vi "Read.vi"(8 "error in (no error)":errorcluster, 10 "count":i32, 11 "Stream Upload Controller in":refnum<class "Stream Upload Controller.lvclass">) -> (0 "error out":errorcluster, 2 "data":u8[](array[numeric]), 3 "Stream Upload Controller out":refnum<class "Stream Upload Controller.lvclass">)   [LabVIEW 2020, in "NI_SFTP.lvlib" / "Stream Upload Controller.lvclass"]
uses:
  <vilib>/net/SFTP/API/Support/Upload/Stream/Stream Upload Controller.lvclass
  <vilib>/net/SFTP/API/Support/Upload/Stream/Stream Upload Controller.lvclass/Stream Upload Controller.ctl
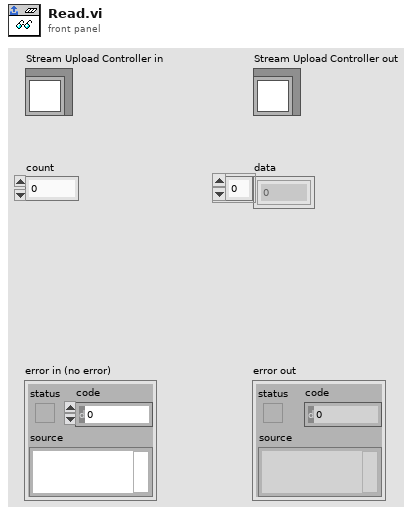
[diagram p1: front panel]
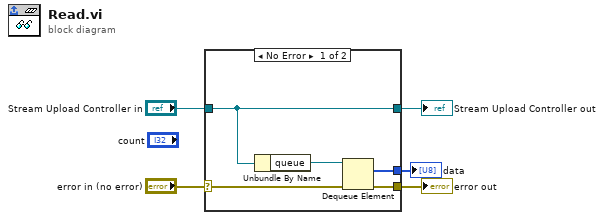
[diagram p0: block diagram]
diagram:
  n1 = case shown="No Error" "error in (no error)" {
    selector: "error in (no error)" -> [w7 w12]
    tunnel: [w6 w12] -> w4
    tunnel: [w10 w11] -> w2
    tunnel: "Stream Upload Controller in" -> [w10 w11]
    tunnel: [w8 _] -> w1
    frame No Error {
      n2 = Unbundle By Name(w10) -> ("queue"=w9:refnum<queue>)
      n3 = Dequeue Element(queue=w9, error in (no error)=w7) -> (element=w8:u8[], error out=w6:errorcluster)  [unwired: 1 in, 2 out]
    }
    frame Error {
    }
  }
  "error out" <- w4
  "Stream Upload Controller out" <- w2
  "data" <- w1
